vi "Get SMO HELP getAll.vi"(8 "error in (no error)":errorcluster, 11 "Instrument.Lockin in":refnum<class "Instrument.Lockin.lvclass">) -> (0 "error out":errorcluster, 2 "response cluster":variant, 3 "Instrument.Lockin out":refnum<class "Instrument.Lockin.lvclass">)   [LabVIEW 2019, in "Instrument.Lockin.lvlib" / "Instrument.Lockin.lvclass"]
uses:
  Instrument.Lockin.lvclass
  Typedefs/Lockin.getAllData--Cluster.ctl
  Instrument.DAQ/Typedefs/Status--enum.ctl
  Instrument.DAQ/Typedefs/PublicEvents--DAQ.getWaveforms.ctl
  Instrument.DAQ/Typedefs/Results--Cluster.ctl
  Instrument.DAQ/Typedefs/PublicEvents--DAQ.getSweepWaveforms.ctl
  <userlib>/LevyLab/Instrument Framework/Instrument Types/Lockin/Instrument.LockinAPI.lvclass
  Instrument.DAQ/Instrument.DAQ.lvclass
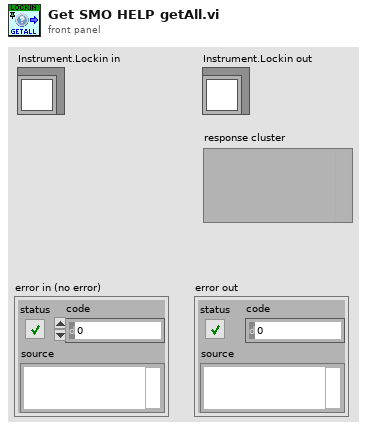
[diagram p1: front panel]
types:
  T1 = typedef "Instrument.Lockin.lvlib/Instrument.Lockin.lvclass/Lockin.getAllData--Cluster.ctl" = cluster{"DAQ State":T2, "Waveforms":T3, "Results":T4, "SweepWaveforms":T5}
  T2 = typedef "Instrument.Lockin.lvlib/Instrument.DAQ.lvclass/Status--enum.ctl" = enum16{"idle", "created", "started", "stopped", "sweeping"}
  T3 = typedef "Instrument.Lockin.lvlib/Instrument.DAQ.lvclass/PublicEvents--DAQ.getWaveforms.ctl" = cluster{"AO":waveform(dbl)[], "AI":waveform(dbl)[], "REF_X":waveform(dbl)[], "REF_Y":waveform(dbl)[], "X":waveform(dbl)[], "Y":waveform(dbl)[]}
  T4 = typedef "Instrument.Lockin.lvlib/Instrument.DAQ.lvclass/Results--Cluster.ctl" = cluster{"Time Stamp":timestamp, "Results (Dictionary)":cluster{"key":string, "value":dbl[]}[]}
  T5 = typedef "Instrument.Lockin.lvlib/Instrument.DAQ.lvclass/PublicEvents--DAQ.getSweepWaveforms.ctl" = cluster{"AO":waveform(dbl)[], "AI":waveform(dbl)[], "X":waveform(dbl)[], "Y":waveform(dbl)[]}
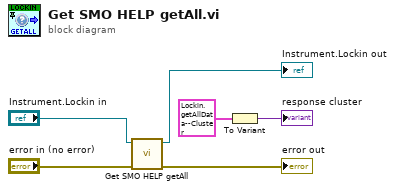
[diagram p0: block diagram]
diagram:
  n1 = call-parent "Get SMO HELP getAll.vi"("error in (no error)"="error in (no error)", "Instrument in"="Instrument.Lockin in") -> ("error out"=→"error out":errorcluster, "Instrument out"=→"Instrument.Lockin out":refnum<class "Instrument.Lockin.lvclass">)  [unwired: 7 in, 1 out]
  n2 = To Variant(anything=T1 {"DAQ State"=enum."idle", "Waveforms"={"AO"=[], "AI"=[], "REF_X"=[], "REF_Y"=[], "X"=[], "Y"=[]}, "Results"={"Time Stamp"=timestamp(0 s since 1904-01-01), "Results (Dictionary)"=[]}, "SweepWaveforms"={"AO"=[], "AI"=[], "X"=[], "Y"=[]}} ("Data")) -> (Variant=→"response cluster":variant)
